vi "Enable Generator Output.vi"(8 "error in (no error)":errorcluster, 9 "Waveform Generator Number (1: Waveform Generator 1)":i32(ring)=1 items=["Waveform Generator 1"=1, "Waveform Generator 2"=2], 10 "Enable Output (F: Disable)":bool, 11 "VISA resource name":refnum<visa-resource-name>) -> (0 "error out":errorcluster, 3 "VISA resource name out":refnum<visa-resource-name>)   [LabVIEW 2015, in "Agilent 2000 3000 X-Series.lvlib"]
doc: "Specifies the output state of waveform generator."
uses:
  <instrlib>/Agilent 2000 3000 X-Series/Agilent 2000 3000 X-Series.lvlib
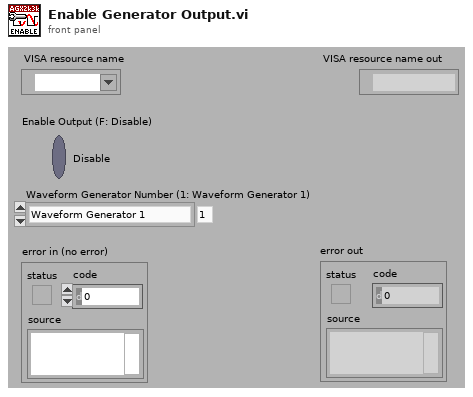
[diagram p1: front panel]
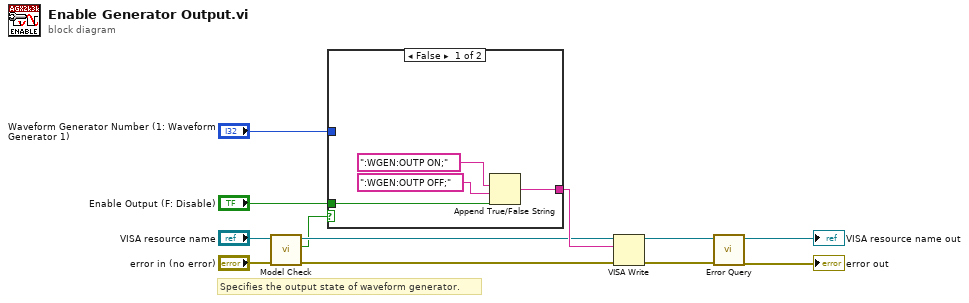
[diagram p0: block diagram]
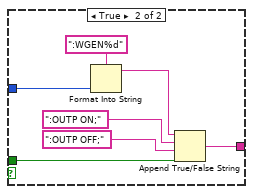
[diagram p2: hidden frame]
diagram:
  # "Specifies the output state of waveform generator."
  n1 = call <instrlib>:"Model Check.vi"("error in (no error)"="error in (no error)", "VISA resource name"="VISA resource name") -> ("error out"=w3:errorcluster, "Not 2000 or 3000 Series"=w2:bool, "VISA resource name out"=w4:refnum<visa-resource-name>)  [unwired: 7 out]
  n2 = case shown="False" w2 {
    tunnel: "Enable Output (F: Disable)" -> [w16 w21]
    tunnel: [w13 w17] -> w11
    tunnel: "Waveform Generator Number (1: Waveform Generator 1)" -> [_ w19]
    frame False {
      n3 = Append True/False String(1:w16, 2:":WGEN:OUTP OFF;", 3:":WGEN:OUTP ON;") -> (0:w13:string)  [unwired: 1 out]
    }
    frame True {
      n4 = Format Into String(format string=":WGEN%d", w19) -> (resulting string=w18:string)  [unwired: 2 in, 1 out]
      n5 = Append True/False String(1:w21, 2:":OUTP OFF;", 3:":OUTP ON;", 4:w18) -> (0:w17:string)
    }
  }
  n6 = VISA Write(VISA resource name=w4, write buffer=w11, error in (no error)=w3) -> (VISA resource name out=w10:refnum<visa-resource-name>, error out=w9:errorcluster)  [unwired: 1 out]
  n7 = call <instrlib>:"Error Query.vi"("error in (no error)"=w9, "VISA resource name"=w10) -> ("error out"=→"error out":errorcluster, "VISA resource name out"=→"VISA resource name out":refnum<visa-resource-name>)  [unwired: 8 out]
